vi "_LazyBoot4.vi"(6 "Variant in":variant, 8 "error in (no error)":errorcluster, 9 "Shift Pressed?":bool, 10 "QD Combo Box Ref":refnum<vi>, 11 "QD Launch VI Ref":refnum<vi>) -> (0 "error out":errorcluster, 4 "Variant out":variant)   [LabVIEW 2014, in "NEVSTOP QD Shortcuts.lvlib"]
uses:
  NEVSTOP QD Shortcuts.lvlib
  <vilib>/SLK/Lazyboots Menu Tool/Library/Lazyboots Menu Tool.lvlib
panel:
  in  "Undo Name":string="lazyboot4"
  # "Do not change the connector pane of this VI.\n\nSee the block diagram for directions on how to use this template."
  # "Specify the name of the Undo transaction"
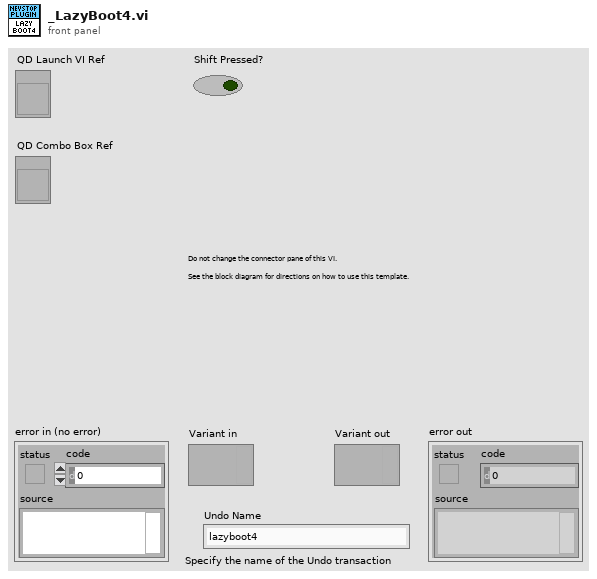
[diagram p1: front panel]
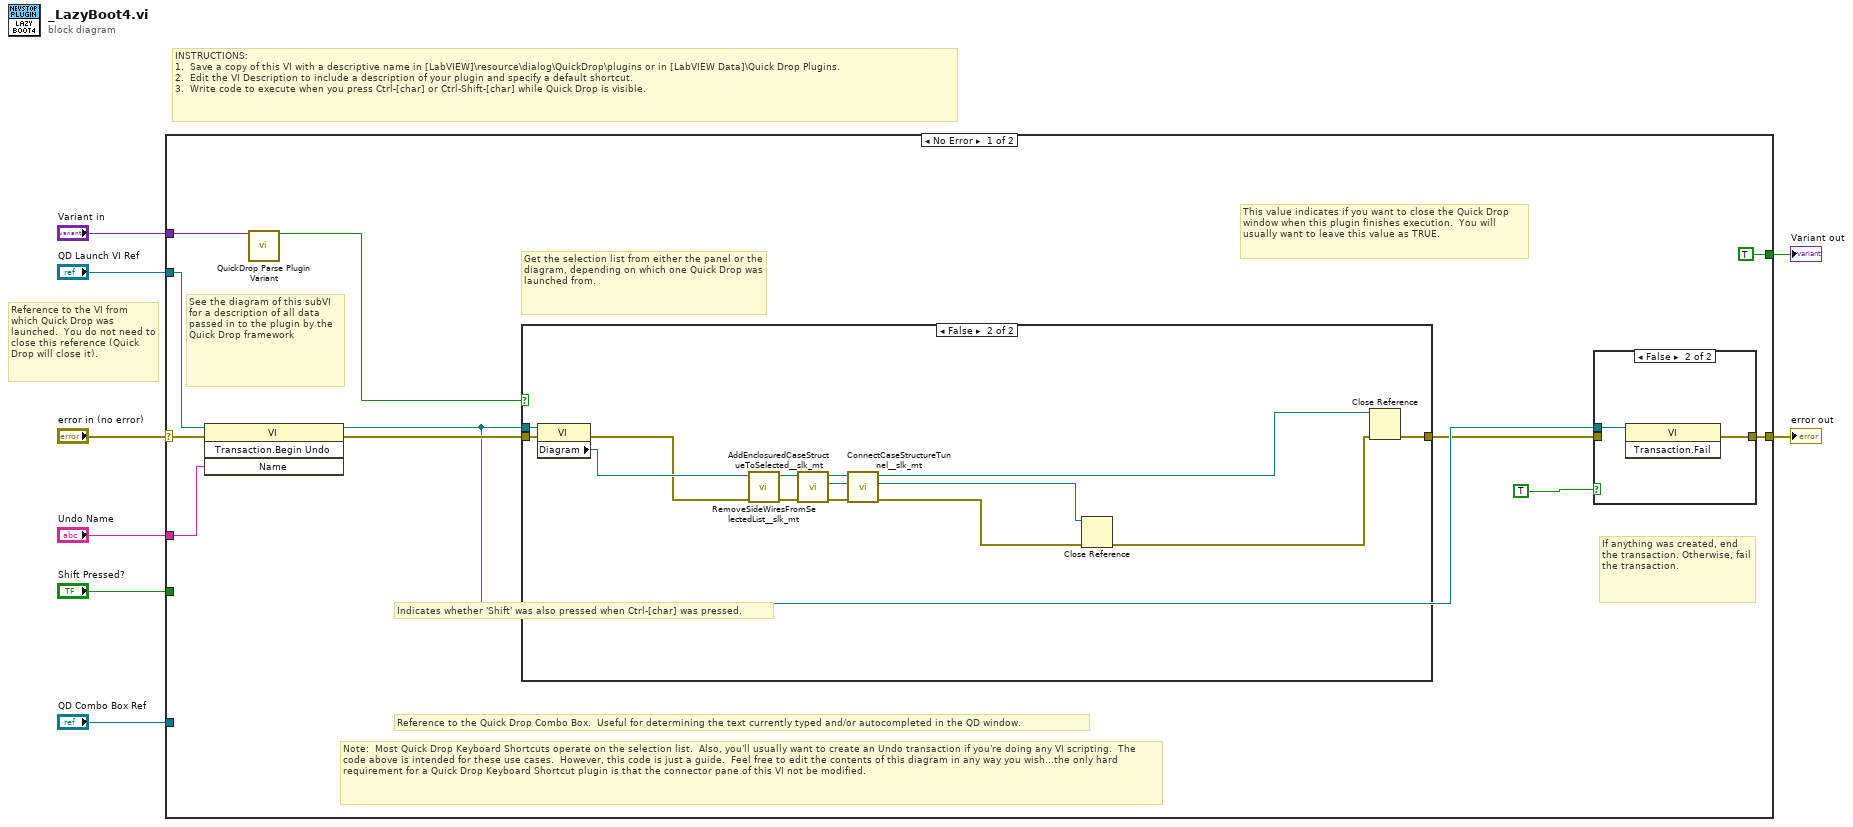
[diagram p0: block diagram]
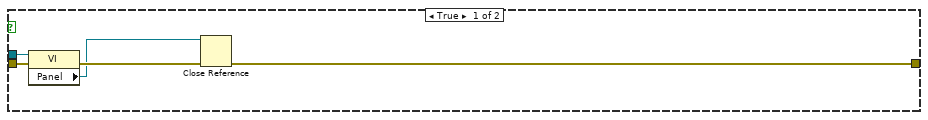
[diagram p2: hidden frame]
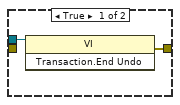
[diagram p3: hidden frame]
diagram:
  # "Reference to the VI from which Quick Drop was launched.  You do not need to close this reference (Quick Drop will close it)."
  # "INSTRUCTIONS:\n1.  Save a copy of this VI with a descriptive name in [LabVIEW]\\resource\\dialog\\QuickDrop\\plugins or in [LabVIEW Data]\\Quick Drop Plugins.\n2.  Edit the VI Description to include a description of your plugin and specify a default shortcut. \n3.  Write code to execute when you press Ctrl-[char] or Ctrl-Shift-[char] while Quick Drop is visible."
  n1 = case shown="No Error" "error in (no error)" {
    selector: "error in (no error)" -> [w18 w43]
    tunnel: [w12 w43] -> w7
    tunnel: "QD Launch VI Ref" -> [w17 _]
    tunnel: "Shift Pressed?" -> [_ _]
    tunnel: "QD Combo Box Ref" -> [_ _]
    tunnel: "Variant in" -> [w19 _]
    tunnel: "Undo Name" -> [w16 _]
    tunnel: [TRUE _] -> w1
    frame No Error {
      # "Get the selection list from either the panel or the diagram, depending on which one Quick Drop was launched from."
      # "This value indicates if you want to close the Quick Drop window when this plugin finishes execution.  You will usually want to leave this value as TRUE."
      # "Indicates whether 'Shift' was also pressed when Ctrl-[char] was pressed."
      # "Note:  Most Quick Drop Keyboard Shortcuts operate on the selection list.  Also, you'll usually want to create an Undo transaction if you're doing any VI scripting.  The code above is intended for these use cases.  However, this code is just a guide.  Feel free to edit the contents of this diagram in any way you wish...the only hard requirement for a Quick Drop Keyboard Shortcut plugin is that the connector pane of this VI not be modified."
      # "If anything was created, end the transaction. Otherwise, fail the transaction."
      # "See the diagram of this subVI for a description of all data passed in to the plugin by the Quick Drop framework"
      # "Reference to the Quick Drop Combo Box.  Useful for determining the text currently typed and/or autocompleted in the QD window."
      n2 = invoke class="VI" method="Transaction.Begin Undo"(reference=w17, error in=w18, "Name"=w16) -> (reference out=w11:refnum<vi>, error out=w13:errorcluster)  [unwired: 1 in, 2 out]
      n3 = call <vilib>:"QuickDrop Parse Plugin Variant.vi"("QDKS Variant in"=w19) -> ("QD Launch VI Panel?"=w14:bool)  [unwired: 12 in, 2 out]
      n4 = case shown="False" w14 {
        tunnel: w13 -> [w24 w38]
        tunnel: w11 -> [w23 w37]
        tunnel: [w20 w28] -> w9
        frame True {
          n5 = property class="VI"(reference=w23, error in=w24) -> (error out=w22:errorcluster, "Panel"=w21:refnum<vi>)  [unwired: 1 out]
          n6 = Close Reference(reference=w21, error in (no error)=w22) -> (error out=w20:errorcluster)
        }
        frame False {
          n7 = property class="VI"(reference=w37, error in=w38) -> (error out=w30:errorcluster, "Diagram"=w31:refnum<vi>)  [unwired: 1 out]
          n8 = call <vilib>:"RemoveSideWiresFromSelectedList__slk_mt.vi"("error in (no error)"=w30, "diagram refnum in"=w31) -> ("error out"=w32:errorcluster, "duplicated diagram refnum out"=w33:refnum<vi>)  [unwired: 8 in]
          n9 = call <vilib>:"AddEnclosuredCaseStructueToSelected__slk_mt.vi"("error in (no error)"=w32, "diagram refnum in"=w33) -> ("error out"=w34:errorcluster, "case structure refnum out"=w35:refnum<vi>, "duplicated diagram refnum out"=w36:refnum<vi>)  [unwired: 7 in]
          n10 = call <vilib>:"ConnectCaseStructureTunnel__slk_mt.vi"("error in (no error)"=w34, "case structure refnum in"=w35, "diagram refnum in"=w36) -> ("error out"=w29:errorcluster, "duplicated case structure refnum out"=w25:refnum<vi>, "duplicated diagram refnum out"=w27:refnum<vi>)  [unwired: 6 in]
          n11 = Close Reference(reference=w25, error in (no error)=w29) -> (error out=w26:errorcluster)
          n12 = Close Reference(reference=w27, error in (no error)=w26) -> (error out=w28:errorcluster)
        }
      }
      n13 = case shown="False" TRUE {
        tunnel: w11 -> [w39 w41]
        tunnel: [w40 w42] -> w12
        tunnel: w9 -> [_ _]
        frame True {
          n14 = invoke class="VI" method="Transaction.End Undo"(reference=w39) -> (error out=w40:errorcluster)  [unwired: 2 in, 2 out]
        }
        frame False {
          n15 = invoke class="VI" method="Transaction.Fail"(reference=w41) -> (error out=w42:errorcluster)  [unwired: 2 in, 2 out]
        }
      }
    }
    frame Error {
    }
  }
  "error out" <- w7
  "Variant out" <- w1
